vi "Write Val.vi"(8 "error in (no error)":errorcluster, 10 "Val":dbl, 11 "DBL STEP in":refnum<class "DBL STEP.lvclass">) -> (0 "error out":errorcluster, 3 "DBL STEP out":refnum<class "DBL STEP.lvclass">)   [LabVIEW 2014, in "Calibration.lvlib" / "DBL STEP.lvclass"]
uses:
  DBL STEP.lvclass
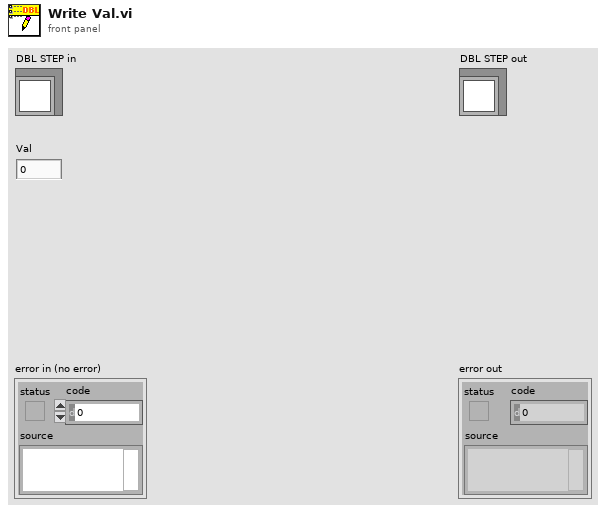
[diagram p1: front panel]
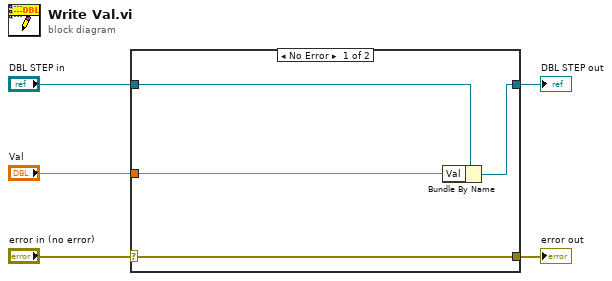
[diagram p0: block diagram]
diagram:
  n1 = case shown="No Error" "error in (no error)" {
    selector: "error in (no error)" -> [w9 w10]
    tunnel: [w9 w10] -> w4
    tunnel: [w7 w11] -> w2
    tunnel: "DBL STEP in" -> [w8 w11]
    tunnel: "Val" -> [w6 _]
    frame No Error {
      n2 = Bundle By Name(cluster=w8, "Val"=w6) -> (w7:refnum<class "DBL STEP.lvclass">)
    }
    frame Error {
    }
  }
  "error out" <- w4
  "DBL STEP out" <- w2
